vi "Get neighbor square.vi"(8 "error in (no error)":errorcluster, 9 "Vector (0, 0)":cluster{i8, i8}, 10 "Neighbor (vector)":T4=enum."vector", 11 "Square in":T1={"File"=enum."d", "Rank"=enum."4"}) -> (0 "error out":errorcluster, 2 "Valid":bool, 3 "Square out":T1={"File"=enum."d", "Rank"=enum."4"})   [LabVIEW 2016, in "Chesslib.lvlib"]
uses:
  Chesslib.lvlib
  typedef/Square.ctl
  typedef/File.ctl
  typedef/Rank.ctl
  typedef/Neighbor.ctl
  <vilib>/Utility/error.llb/Error Cluster From Error Code.vi
  <vilib>/ErrorRing/Error Ring.xnode
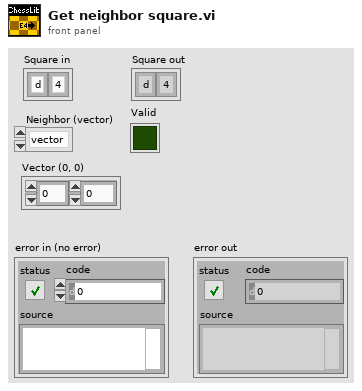
[diagram p1: front panel]
types:
  T1 = typedef "Chesslib.lvlib/Square.ctl" = cluster{"File":T2, "Rank":T3}
  T2 = typedef "Chesslib.lvlib/File.ctl" = enum8{"a", "b", "c", "d", "e", "f", "g", "h"}
  T3 = typedef "Chesslib.lvlib/Rank.ctl" = enum8{"1", "2", "3", "4", "5", "6", "7", "8"}
  T4 = typedef "Chesslib.lvlib/Neighbor.ctl" = enum16{"N", "NW", "W", "SW", "S", "SE", "E", "NE", "vector"}
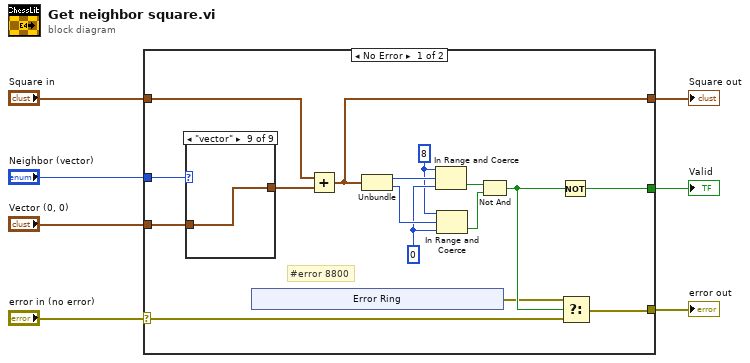
[diagram p0: block diagram]
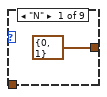
[diagram p2: hidden frame]
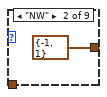
[diagram p3: hidden frame]
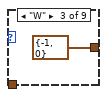
[diagram p4: hidden frame]
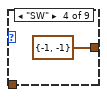
[diagram p5: hidden frame]
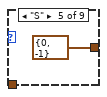
[diagram p6: hidden frame]
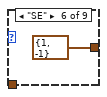
[diagram p7: hidden frame]
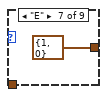
[diagram p8: hidden frame]
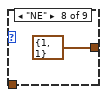
[diagram p9: hidden frame]
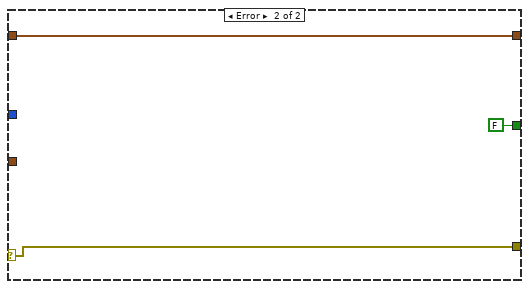
[diagram p10: hidden frame]
diagram:
  n1 = case shown="No Error" "error in (no error)" {
    selector: "error in (no error)" -> [w11 w40]
    tunnel: "Neighbor (vector)" -> [w23 _]
    tunnel: "Square in" -> [w21 w39]
    tunnel: [w9 w39] -> w5
    tunnel: "Vector (0, 0)" -> [w14 _]
    tunnel: [w13 w40] -> w3
    tunnel: [w10 FALSE] -> w1
    frame No Error {
      w17 = u8 8 ("lower limit")
      w18 = u8 0 ("lower limit")
      # "#error 8800"
      n2 = case shown="\"vector\"" w23 {
        tunnel: [cluster{i8, i8} {0, 1} cluster{i8, i8} {-1, 1} cluster{i8, i8} {-1, 0} cluster{i8, i8} {-1, -1} cluster{i8, i8} {0, -1} cluster{i8, i8} {1, -1} cluster{i8, i8} {1, 0} cluster{i8, i8} {1, 1} w37] -> w22
        tunnel: w14 -> [_ _ _ _ _ _ _ _ w37]
        frame "N" {
        }
        frame "NW" {
        }
        frame "W" {
        }
        frame "SW" {
        }
        frame "S" {
        }
        frame "SE" {
        }
        frame "E" {
        }
        frame "NE" {
        }
        frame "vector" {
        }
      }
      n3 = xnode "Error Ring"() -> ("error out"=w8:errorcluster)
      n4 = Add(x=w21, y=w22) -> (x+y=w9:cluster{u8, u8})
      n5 = Unbundle(w9) -> (w20:u8, w19:u8)
      n6 = In Range and Coerce(upper limit=w17, x=w20, lower limit=w18) -> (In Range?=w16:bool)  [unwired: 1 out]
      n7 = In Range and Coerce(upper limit=w17, x=w19, lower limit=w18) -> (In Range?=w15:bool)  [unwired: 1 out]
      n8 = Not And(1:w15, 2:w16) -> (0:w12:bool)
      n9 = Not(x=w12) -> (.not. x?=w10:bool)
      n10 = Select(t=w8, s=w12, f=w11) -> (s? t:f=w13:errorcluster)
    }
    frame Error {
    }
  }
  "Square out" <- w5
  "Valid" <- w1
  "error out" <- w3
